vi "n set pixel line.vi"(6 "dy":dbl, 7 "dx":dbl, 8 "error in (no error)":errorcluster, 9 "pixelperiod":u16, 10 "pixelmode":u16, 11 "n":u16) -> (0 "error out":errorcluster)   [LabVIEW 2015, in "SCANalone4x64.lvlib"]
doc: "__declspec(dllimport) void __stdcall n_set_pixel_line(unsigned short n, unsigned short pixelmode, unsigned short pixelperiod, double dx, double dy);"
uses:
  <userlib>/SCANalone4x64/SCANalone4x64.lvlib
  <userlib>/SCANalone4x64/SCANalone4x64.dll
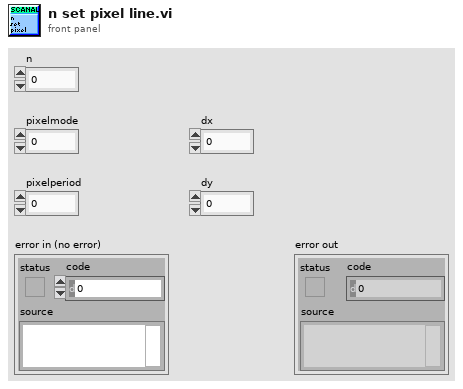
[diagram p1: front panel]
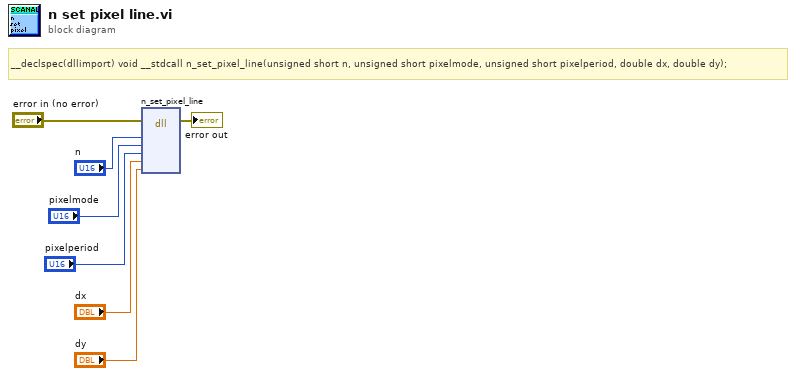
[diagram p0: block diagram]
diagram:
  # "__declspec(dllimport) void __stdcall n_set_pixel_line(unsigned short n, unsigned short pixelmode, unsigned short pixelperiod, double dx, double dy);"
  n1 = dll-call lib="C:/Program Files/National Instruments/LabVIEW 2015/user.lib/SCANalone4x64/SCANalone4x64.*" fn="n_set_pixel_line"(error in="error in (no error)", "n"="n", "pixelmode"="pixelmode", "pixelperiod"="pixelperiod", "dx"="dx", "dy"="dy") -> (error out=→"error out":errorcluster)  [unwired: 8 in, 1 out]
